vi "DMM Configuration.vi"(8 "error in (no error)":errorcluster, 11 "Node Ptr":T1 format="%.0x") -> (0 "error out":errorcluster)   [LabVIEW 2016, in "DMM-SWITCH-ScanList System Explorer.lvlib"]
uses:
  DMM-SWITCH-ScanList System Explorer.lvlib
  <vilib>/NI Veristand/Custom Device API/Custom Device Item Ref.ctl
  Configuration Controls/DMM Temp.ctl
  <instrlib>/niDMM/nidmm.llb/niDMM Transducer Type.ctl
  <instrlib>/niDMM/nidmm.llb/niDMM Thermocouple Type.ctl
  <instrlib>/niDMM/nidmm.llb/niDMM RTD Type.ctl
  <instrlib>/niDMM/nidmm.llb/niDMM Thermistor Type.ctl
  <instrlib>/niDMM/nidmm.llb/niDMM Function.ctl
  Shared/Constants.vi
  <vilib>/NI Veristand/Custom Device API/Get Item Property (U16).vi
  <vilib>/NI Veristand/Custom Device API/Get Item Property (Double).vi
  <vilib>/NI Veristand/Custom Device API/Get Item Property (String).vi
  <vilib>/NI Veristand/Custom Device API/Get Item Property (Variant).vi
  <vilib>/NI Veristand/Custom Device API/Set Item Property (String).vi
  <vilib>/NI Veristand/Custom Device API/Set Item Property (Double).vi
  <vilib>/NI Veristand/Custom Device API/Set Item Property (Variant).vi
  <vilib>/NI Veristand/Custom Device API/Set Item Property (U16).vi
  <vilib>/NI Veristand/Custom Device API/Custom Device API.lvlib
  Shared/DMM-SWITCH-ScanList Shared.lvlib
panel:
  in  "Temp3":dbl
  in  "Temp2":u16(ring)
  in  "Transducer":u16(ring)
  in  "Range":u16(ring)
  in  "Resolution in Digits":u16(ring)
  in  "Measurements":u16(ring)
  in  "DMM Resource Name":string
  in  "Header":cluster{"Section Name":string}={"Section Name"="Custom Device Item Settings"}
  in  "Description":string
  in  "Name":string
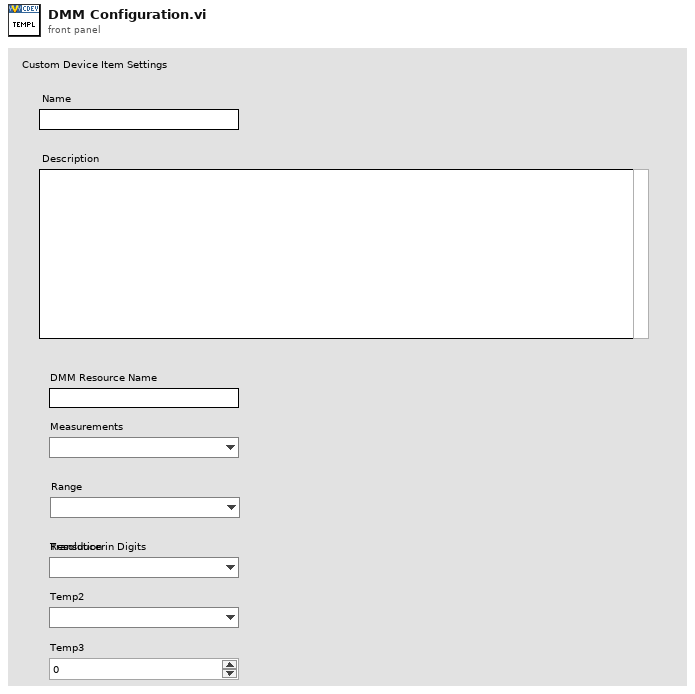
[diagram p1: front panel]
types:
  T1 = typedef "Custom Device API.lvlib/Custom Device Item Ref.ctl" = u64
  T2 = typedef "DMM-SWITCH-ScanList System Explorer.lvlib/DMM Temp.ctl" = cluster{"DMM Temp - Transducer Type":T3, "DMM Temp - Thermocouple Type":T4, "DMM Temp - Fixed Reference Junction":dbl, "DMM Temp - RTD Type":T5, "DMM Temp - RTD Resistance":dbl, "DMM Temp - Thermistor Type":T6, "DMM Temp - RTD A":dbl, "DMM Temp - RTD B":dbl, "DMM Temp - RTD C":dbl, "DMM Temp - Thermistor A":dbl, "DMM Temp - Thermistor B":dbl, "DMM Temp - Thermistor C":dbl}
  T3 = typedef "niDMM Transducer Type.ctl" = i32
  T4 = typedef "niDMM Thermocouple Type.ctl" = i32
  T5 = typedef "niDMM RTD Type.ctl" = enum16{"Custom", "Pt3750", "Pt3851", "Pt3911", "Pt3916", "Pt3920", "Pt3928"}
  T6 = typedef "niDMM Thermistor Type.ctl" = enum16{"Custom", "44004", "44006", "44007"}
  T7 = typedef "Custom Device API.lvlib/Custom Device Item Info.ctl" = cluster{"Name":string, "Is Channel":bool, "GUID":string, "Is Waveform":bool}
  T8 = cluster{"Measurements":refnum<vi>, "Range":refnum<vi>, "Resolution in Digits":refnum<vi>, "Transducer":refnum<vi>, "Temp2":refnum<vi>, "Temp3":refnum<vi>}
  T9 = typedef "niDMM Function.ctl" = enum16{"DC Volts", "AC Volts", "DC Current", "AC Current", "2-wire Resistance", "4-wire Resistance", "Diode", "Frequency", "Period", "AC Volts DC Coupled", "Capacitance", "Inductance", "Temperature"}
  T10 = typedef "Custom Device API.lvlib/Custom Device Commands.ctl" = enum16{"Default", "Item renamed", "Shutdown", "Dynamic button pressed"}
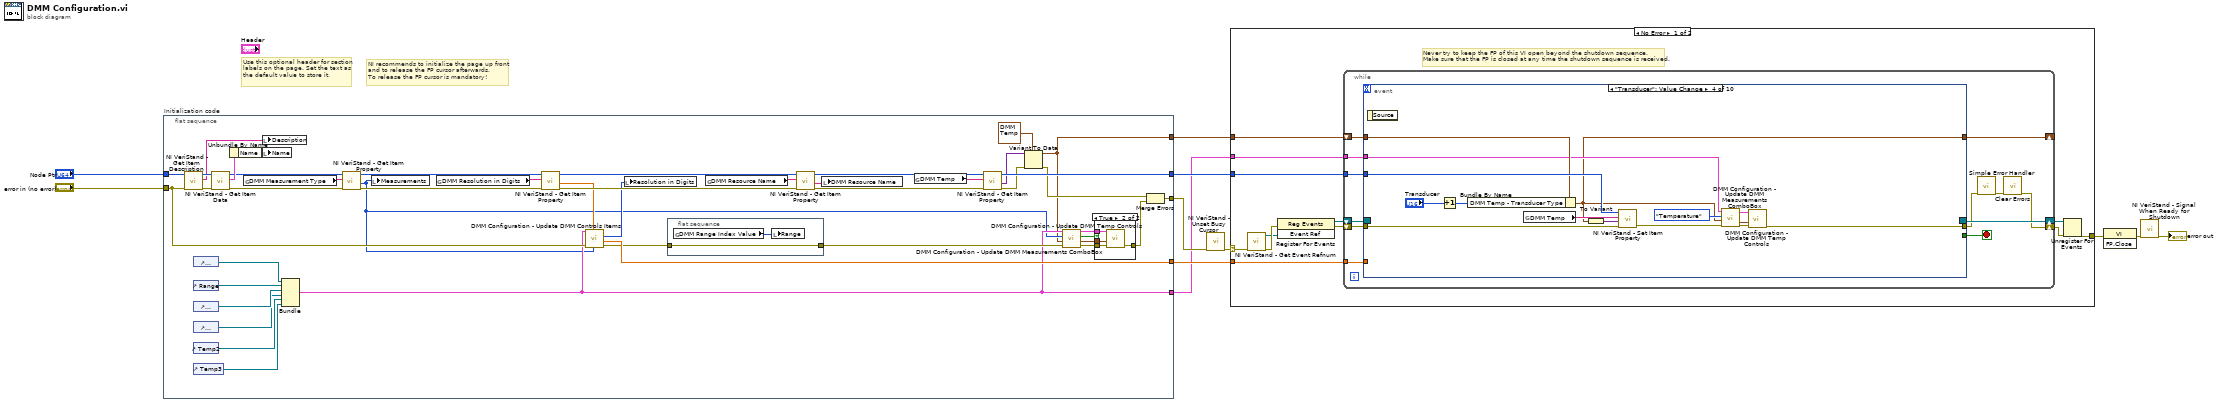
[diagram p0: block diagram]
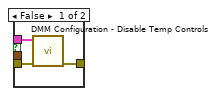
[diagram p2: hidden frame]
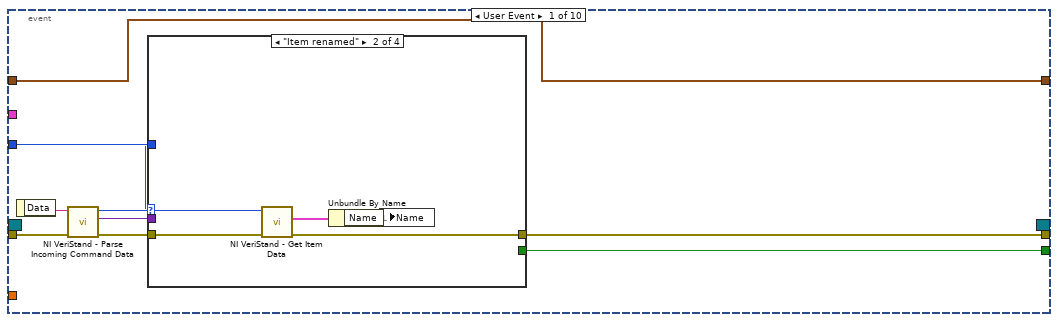
[diagram p3: hidden frame]
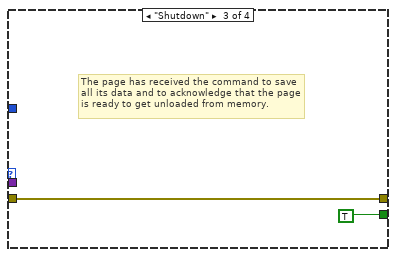
[diagram p5: hidden frame]
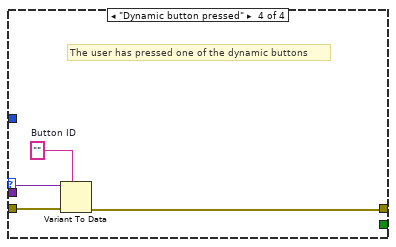
[diagram p6: hidden frame]
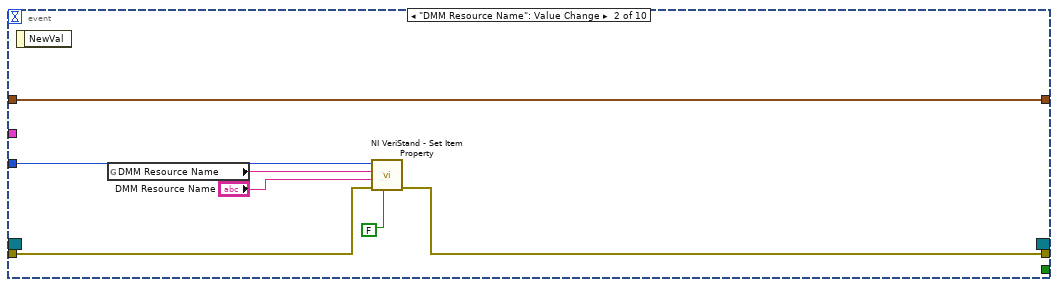
[diagram p7: hidden frame]
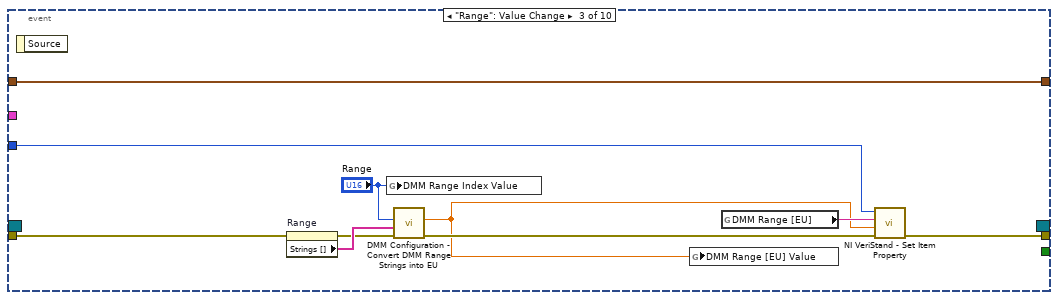
[diagram p8: hidden frame]
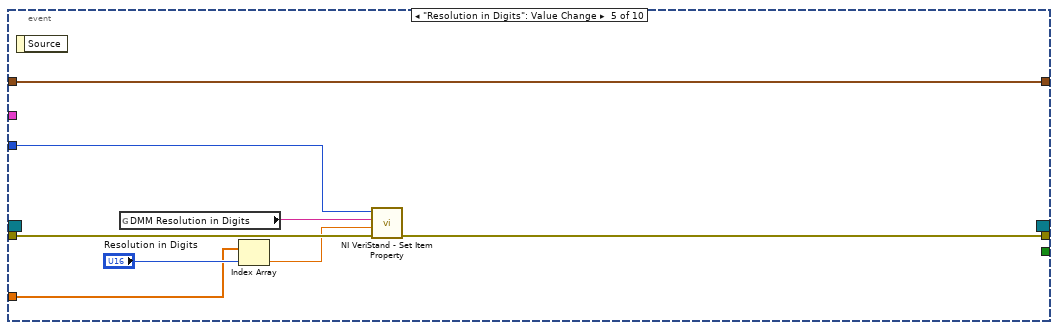
[diagram p9: hidden frame]
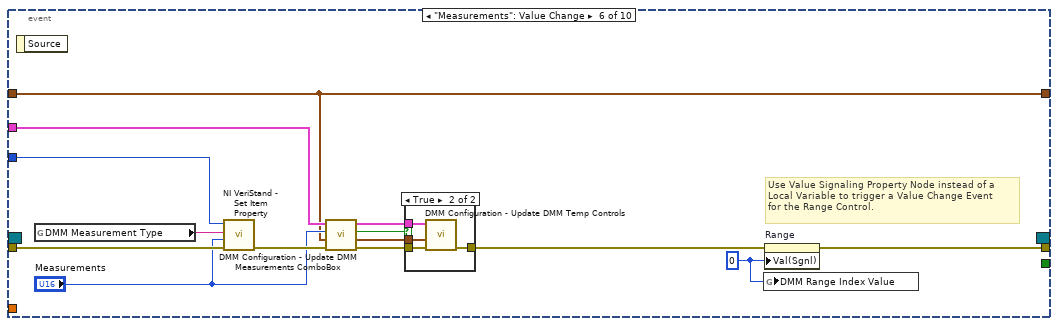
[diagram p10: hidden frame]
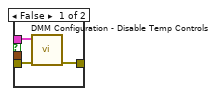
[diagram p11: hidden frame]
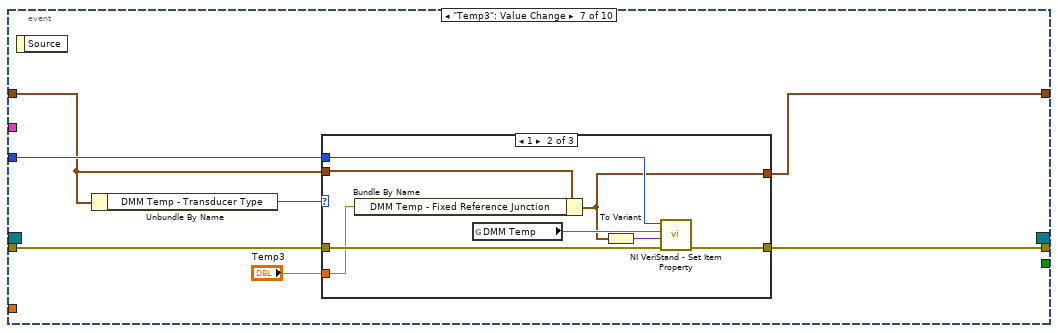
[diagram p12: hidden frame]
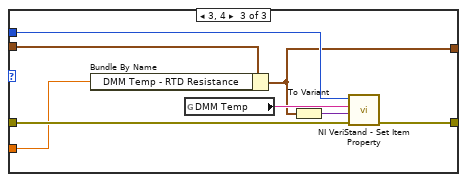
[diagram p14: hidden frame]
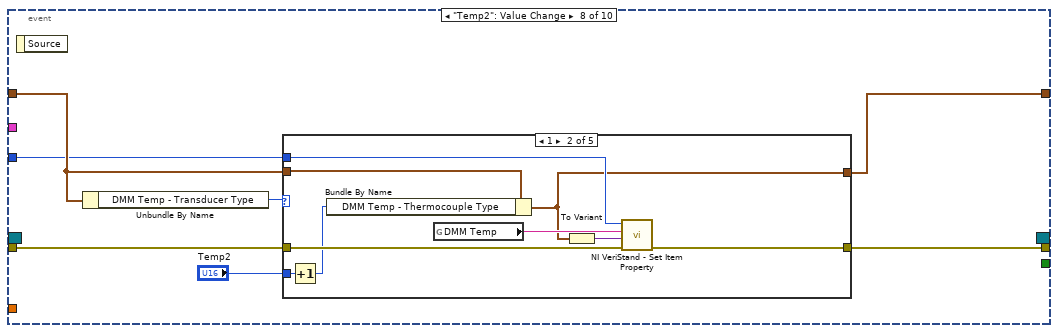
[diagram p15: hidden frame]
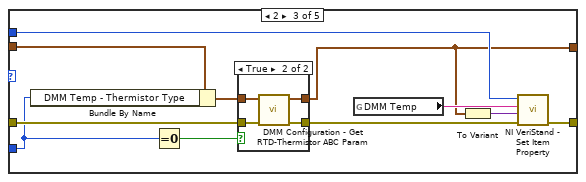
[diagram p17: hidden frame]
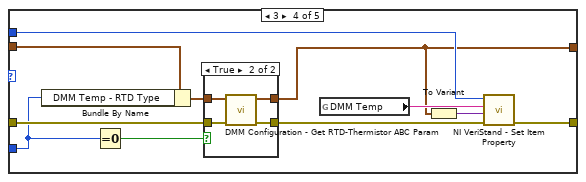
[diagram p19: hidden frame]
diagram:
  # "Use this optional header for section labels on the page. Set the text as the default value to store it."
  # "NI recommends to initialize the page up front\nand to release the FP cursor afterwards.\nTo release the FP cursor is mandatory!"
  n1 = flat-sequence "Initialization code" {
    tunnel: "error in (no error)" -> [w39]
    tunnel: "Node Ptr" -> [w55]
    tunnel: [w43] -> w7
    tunnel: [w25] -> w4
    tunnel: [w36] -> w3
    tunnel: [w17] -> w2
    tunnel: [w13] -> w1
    frame #0 {
      n2 = call <vilib>:"NI VeriStand - Get Item Description.vi"("error in (no error)"=w39, "Item Ref in"=w55) -> ("error out"=w53:errorcluster, "Description"=w54:string, "Item Ref out"=w56:T1)  [unwired: 7 out]
      n3 = control-ref of="Measurements"() -> (w29:refnum<vi>)
      n4 = control-ref of="Range"() -> (w34:refnum<vi>)
      n5 = control-ref of="Resolution in Digits"() -> (w33:refnum<vi>)
      n6 = control-ref of="Transducer"() -> (w31:refnum<vi>)
      n7 = control-ref of="Temp2"() -> (w30:refnum<vi>)
      n8 = control-ref of="Temp3"() -> (w32:refnum<vi>)
      n9 = call <vilib>:"NI VeriStand - Get Item Data.vi"("error in (no error)"=w53, "Item Ref in"=w56) -> ("error out"=w50:errorcluster, "Item Info"=w52:T7, "Item Ref out"=w49:T1)  [unwired: 7 out]
      n10 = Unbundle By Name(w52) -> ("Name"=w51:string)
      n11 = global read "Constants.vi" "DMM Measurement Type"() -> (w42:string)
      n12 = local write "Description"(w54) -> ()
      n13 = local write "Name"(w51) -> ()
      n14 = Bundle("Measurements"=w29, "Range"=w34, "Resolution in Digits"=w33, "Transducer"=w31, "Temp2"=w30, "Temp3"=w32) -> (w17:T8)  [unwired: 1 in]
      n15 = call-poly <vilib>:"NI VeriStand - Get Item Property.vi"("error in (no error)"=w50, "Property Name"=w42, "Item Ref in"=w49) -> ("error out"=w47:errorcluster, "Value"=w14:u16, "Item Ref out"=w48:T1)  [unwired: 5 in, 1 out]
      n16 = local write "Measurements"(w14) -> ()
      n17 = global read "Constants.vi" "DMM Resolution in Digits"() -> (w45:string)
      n18 = call-poly <vilib>:"NI VeriStand - Get Item Property.vi"("error in (no error)"=w47, "Property Name"=w45, "Item Ref in"=w48) -> ("error out"=w41:errorcluster, "Value"=w38:dbl, "Item Ref out"=w40:T1)  [unwired: 5 in, 1 out]
      n19 = call "DMM Configuration - Update DMM Controls Items.vi"("Measurement In"=w14, "Resolution in Digits Saved Value"=w38, "error in (no error)"=w39, "Measurement Controls Refs"=w17) -> ("error out"=w35:errorcluster, "Resolution in Digits Array Out"=w36:dbl[], "Resolution in Digits Index"=w37:i32)  [unwired: 5 in]
      n20 = local write "Resolution in Digits"(w37) -> ()
      n21 = flat-sequence {
        tunnel: w35 -> [w64]
        tunnel: [w64] -> w20
        frame #0 {
          n22 = global read "Constants.vi" "DMM Range Index Value"() -> (w65:u16)
          n23 = local write "Range"(w65) -> ()
        }
      }
      n24 = global read "Constants.vi" "DMM Resource Name"() -> (w44:string)
      n25 = call-poly <vilib>:"NI VeriStand - Get Item Property.vi"("error in (no error)"=w41, "Property Name"=w44, "Item Ref in"=w40) -> ("error out"=w27:errorcluster, "Value"=w46:string, "Item Ref out"=w26:T1)  [unwired: 5 in, 1 out]
      n26 = local write "DMM Resource Name"(w46) -> ()
      n27 = global read "Constants.vi" "DMM Temp"() -> (w28:string)
      n28 = call-poly <vilib>:"NI VeriStand - Get Item Property.vi"("error in (no error)"=w27, "Property Name"=w28, "Item Ref in"=w26) -> ("error out"=w24:errorcluster, "Value"=w22:variant, "Item Ref out"=w25:T1)  [unwired: 5 in, 1 out]
      n29 = Variant To Data(error in=w24, type=T2 {"DMM Temp - Transducer Type"=1, "DMM Temp - Thermocouple Type"=6, "DMM Temp - Fixed Reference Junction"=25.0, "DMM Temp - RTD Type"=enum."Pt3851", "DMM Temp - RTD Resistance"=100.0, "DMM Temp - Thermistor Type"=enum."44006", "DMM Temp - RTD A"=0.0039083, "DMM Temp - RTD B"=-5.775e-07, "DMM Temp - RTD C"=-4.183e-12, "DMM Temp - Thermistor A"=0.0010295, "DMM Temp - Thermistor B"=0.0002391, "DMM Temp - Thermistor C"=1.568e-07} ("DMM Temp - Value"), Variant=w22) -> (data=w13:T2, error out=w21:errorcluster)
      n30 = call "DMM Configuration - Update DMM Measurements ComboBox.vi"("error in (no error)"=w20, "DMM Temp - Value In"=w13, "Measurement In"=w14, "Measurement Controls Refs In"=w17) -> ("error out"=w19:errorcluster, "DMM Temp - Value Out"=w12:T2, "Temp Meas?"=w16:bool, "Measurement Controls Refs Out"=w15:T8)  [unwired: 4 in]
      n31 = case shown="True" w16 {
        tunnel: w15 -> [w59 w63]
        tunnel: w12 -> [_ w62]
        tunnel: w19 -> [w58 w61]
        tunnel: [w57 w60] -> w18
        frame False {
          n32 = call "DMM Configuration - Disable Temp Controls.vi"("error in (no error)"=w58, "Measurement Controls Refs"=w59) -> ("error out"=w57:errorcluster)  [unwired: 9 in]
        }
        frame True {
          n33 = call "DMM Configuration - Update DMM Temp Controls.vi"("error in (no error)"=w61, "DMM Temp - Value"=w62, "Measurement Controls Refs"=w63) -> ("error out"=w60:errorcluster)  [unwired: 8 in]
        }
      }
      n34 = Merge Errors(w21, w18) -> (w43:errorcluster)
    }
  }
  n35 = call <vilib>:"NI VeriStand - Unset Busy Cursor.vi"("error in (no error)"=w7) -> ("error out"=w6:errorcluster)  [unwired: 10 out]
  n36 = case shown="No Error" w6 {
    selector: w6 -> [w69 w278]
    tunnel: [w74 w276] -> w11
    tunnel: w4 -> [w70 _]
    tunnel: w3 -> [w68 _]
    tunnel: w2 -> [w67 _]
    tunnel: w1 -> [w66 _]
    frame No Error {
      # "Never try to keep the FP of this VI open beyond the shutdown sequence.\nMake sure that the FP is closed at any time the shutdown sequence is received."
      n37 = call <vilib>:"NI VeriStand - Get Event Refnum.vi"("error in (no error)"=w69) -> ("error out"=w77:errorcluster, "Event Ref"=w73:refnum<user-event>)  [unwired: 9 out]
      n38 = register-events(error in=w77, w73) -> (reference out=w71:refnum<event-registration>, error out=w72:errorcluster)  [unwired: 1 in]
      n39 = while {
        tunnel: w70 -> [w85]
        shift-right: [w82] -> w75
        shift-left: w72 -> [w88]
        shift-right: [w89] -> w76
        shift-left: w71 -> [w87]
        tunnel: w68 -> [w81]
        tunnel: w67 -> [w80]
        shift-right: [w78] -> _
        shift-left: w66 -> [w79]
        stop <- w86 stop-if-true
        n40 = event shown="[3] \"Transducer\": Value Change" {
          selector: w87 -> [_ _ _ _ _ _ _ _ _ _]
          dyn-events: [_ _ _ _ _ _ _ _ _ _] -> w89
          timeout: _ -> [_ _ _ _ _ _ _ _ _ _]
          tunnel: w88 -> [w98 w116 w125 w141 w149 w164 w178 w200 w270 w274]
          tunnel: [w94 _ _ _ _ _ _ _ _ _] -> w86
          tunnel: [w93 w115 w127 w137 w148 w161 w177 w199 w269 w273] -> w84
          tunnel: w85 -> [w92 w117 w124 w140 w150 w159 w175 w201 w268 w275]
          tunnel: w81 -> [_ _ _ _ w144 _ _ _ _ _]
          tunnel: w80 -> [_ _ _ w134 _ w157 _ _ _ _]
          tunnel: w79 -> [w90 w111 w118 w139 w143 w152 w173 w203 w266 w271]
          tunnel: [w90 w111 w118 w129 w143 w152 w172 w198 w266 w271] -> w78
          event User Event {
            n41 = event-data() -> ("Data"=w97:string)  [unwired: 1 out]
            n42 = call <vilib>:"NI VeriStand - Parse Incoming Command Data.vi"("error in (no error)"=w98, "Incoming data"=w97) -> ("error out"=w96:errorcluster, "Outgoing data"=w91:variant, "Action"=w95:T10)  [unwired: 7 out]
            n43 = case shown="\"Item renamed\"" w95 {
              tunnel: w96 -> [w99 w104 w105 w110]
              tunnel: [_ _ TRUE _] -> w94
              tunnel: [w99 w101 w105 w107] -> w93
              tunnel: w92 -> [_ w103 _ _]
              tunnel: w91 -> [_ _ _ w109]
              frame "Default", Default {
              }
              frame "Item renamed" {
                n44 = call <vilib>:"NI VeriStand - Get Item Data.vi"("error in (no error)"=w104, "Item Ref in"=w103) -> ("error out"=w101:errorcluster, "Item Info"=w102:T7)  [unwired: 8 out]
                n45 = Unbundle By Name(w102) -> ("Name"=w100:string)
                n46 = local write "Name"(w100) -> ()
              }
              frame "Shutdown" {
                # "The page has received the command to save all its data and to acknowledge that the page is ready to get unloaded from memory."
              }
              frame "Dynamic button pressed" {
                w108 = ""  # Button ID
                # "The user has pressed one of the dynamic buttons"
                n47 = Variant To Data(error in=w110, type=w108, Variant=w109) -> (error out=w107:errorcluster)  [unwired: 1 out]
              }
            }
          }
          event "DMM Resource Name": Value Change {
            n48 = event-data() -> ()  [unwired: 2 out]
            n49 = global read "Constants.vi" "DMM Resource Name"() -> (w112:string)
            n50 = call-poly <vilib>:"NI VeriStand - Set Item Property.vi"("Binary String (T)"=FALSE, "error in (no error)"=w116, "Value"="DMM Resource Name", "Property Name"=w112, "Item Ref in"=w117) -> ("error out"=w115:errorcluster)  [unwired: 4 in, 2 out]
          }
          event "Range": Value Change {
            n51 = event-data() -> ()  [unwired: 2 out]
            n52 = property on="Range" class="Ring (strict)"(error in=w125) -> (error out=w121:errorcluster, "Strings []"=w122:string[])  [unwired: 1 in, 1 out]
            n53 = global write "Constants.vi" "DMM Range Index Value"("Range") -> ()
            n54 = call "DMM Configuration - Convert DMM Range Strings into EU.vi"("error in (no error)"=w121, "DMM Range ComboBox Strings"=w122, "Dmm Range Index In"="Range") -> ("error out"=w120:errorcluster, "DMM Range [EU]"=w119:dbl)  [unwired: 7 in]
            n55 = global write "Constants.vi" "DMM Range [EU] Value"(w119) -> ()
            n56 = global read "Constants.vi" "DMM Range [EU]"() -> (w126:string)
            n57 = call-poly <vilib>:"NI VeriStand - Set Item Property.vi"("error in (no error)"=w120, "Value"=w119, "Property Name"=w126, "Item Ref in"=w124) -> ("error out"=w127:errorcluster)  [unwired: 5 in, 2 out]
          }
          event "Transducer": Value Change {
            n58 = event-data() -> ()  [unwired: 2 out]
            n59 = Increment(x="Transducer") -> (x+1=w135:u16)
            n60 = Bundle By Name(cluster=w139, "DMM Temp - Transducer Type"=w135) -> (w129:T2)
            n61 = global read "Constants.vi" "DMM Temp"() -> (w142:string)
            n62 = To Variant(anything=w129) -> (Variant=w138:variant)
            n63 = call-poly <vilib>:"NI VeriStand - Set Item Property.vi"("error in (no error)"=w141, "Value"=w138, "Property Name"=w142, "Item Ref in"=w140) -> ("error out"=w131:errorcluster)  [unwired: 5 in, 2 out]
            n64 = call "DMM Configuration - Update DMM Measurements ComboBox.vi"("error in (no error)"=w131, "DMM Temp - Value In"=w129, "Measurement In"=niDMM_Function."Temperature", "Measurement Controls Refs In"=w134) -> ("error out"=w130:errorcluster, "DMM Temp - Value Out"=w128:T2, "Measurement Controls Refs Out"=w133:T8)  [unwired: 4 in, 1 out]
            n65 = call "DMM Configuration - Update DMM Temp Controls.vi"("error in (no error)"=w130, "DMM Temp - Value"=w128, "Measurement Controls Refs"=w133) -> ("error out"=w137:errorcluster)  [unwired: 8 in]
          }
          event "Resolution in Digits": Value Change {
            n66 = event-data() -> ()  [unwired: 2 out]
            n67 = global read "Constants.vi" "DMM Resolution in Digits"() -> (w147:string)
            n68 = Index Array(array=w144, index="Resolution in Digits") -> (element=w146:dbl)
            n69 = call-poly <vilib>:"NI VeriStand - Set Item Property.vi"("error in (no error)"=w149, "Value"=w146, "Property Name"=w147, "Item Ref in"=w150) -> ("error out"=w148:errorcluster)  [unwired: 5 in, 2 out]
          }
          event "Measurements": Value Change {
            w162 = 0
            # "Use Value Signaling Property Node instead of a \nLocal Variable to trigger a Value Change Event \nfor the Range Control."
            n70 = event-data() -> ()  [unwired: 2 out]
            n71 = global read "Constants.vi" "DMM Measurement Type"() -> (w163:string)
            n72 = call-poly <vilib>:"NI VeriStand - Set Item Property.vi"("error in (no error)"=w164, "Value"="Measurements", "Property Name"=w163, "Item Ref in"=w159) -> ("error out"=w160:errorcluster)  [unwired: 5 in, 2 out]
            n73 = call "DMM Configuration - Update DMM Measurements ComboBox.vi"("error in (no error)"=w160, "DMM Temp - Value In"=w152, "Measurement In"="Measurements", "Measurement Controls Refs In"=w157) -> ("error out"=w156:errorcluster, "DMM Temp - Value Out"=w151:T2, "Temp Meas?"=w154:bool, "Measurement Controls Refs Out"=w153:T8)  [unwired: 4 in]
            n74 = case shown="True" w154 {
              tunnel: w153 -> [w165 w171]
              tunnel: w151 -> [_ w170]
              tunnel: w156 -> [w167 w169]
              tunnel: [w166 w168] -> w155
              frame False {
                n75 = call "DMM Configuration - Disable Temp Controls.vi"("error in (no error)"=w167, "Measurement Controls Refs"=w165) -> ("error out"=w166:errorcluster)  [unwired: 9 in]
              }
              frame True {
                n76 = call "DMM Configuration - Update DMM Temp Controls.vi"("error in (no error)"=w169, "DMM Temp - Value"=w170, "Measurement Controls Refs"=w171) -> ("error out"=w168:errorcluster)  [unwired: 8 in]
              }
            }
            n77 = global write "Constants.vi" "DMM Range Index Value"(w162) -> ()
            n78 = property on="Range" class="Ring (strict)"(error in=w155, "Val(Sgnl)"=w162) -> (error out=w161:errorcluster)  [unwired: 1 in, 1 out]
          }
          event "Temp3": Value Change {
            n79 = event-data() -> ()  [unwired: 2 out]
            n80 = Unbundle By Name(w173) -> ("DMM Temp - Transducer Type"=w176:T3)
            n81 = case shown="1" w176 {
              tunnel: w173 -> [w179 w186 w194]
              tunnel: w175 -> [_ w185 w191]
              tunnel: w178 -> [w180 w184 w193]
              tunnel: [w180 w183 w192] -> w177
              tunnel: "Temp3" -> [_ w182 w190]
              tunnel: [w179 w181 w189] -> w172
              frame 0, Default {
              }
              frame 1 {
                n82 = Bundle By Name(cluster=w186, "DMM Temp - Fixed Reference Junction"=w182) -> (w181:T2)
                n83 = global read "Constants.vi" "DMM Temp"() -> (w188:string)
                n84 = To Variant(anything=w181) -> (Variant=w187:variant)
                n85 = call-poly <vilib>:"NI VeriStand - Set Item Property.vi"("error in (no error)"=w184, "Value"=w187, "Property Name"=w188, "Item Ref in"=w185) -> ("error out"=w183:errorcluster)  [unwired: 5 in, 2 out]
              }
              frame 3, 4 {
                n86 = Bundle By Name(cluster=w194, "DMM Temp - RTD Resistance"=w190) -> (w189:T2)
                n87 = global read "Constants.vi" "DMM Temp"() -> (w196:string)
                n88 = To Variant(anything=w189) -> (Variant=w195:variant)
                n89 = call-poly <vilib>:"NI VeriStand - Set Item Property.vi"("error in (no error)"=w193, "Value"=w195, "Property Name"=w196, "Item Ref in"=w191) -> ("error out"=w192:errorcluster)  [unwired: 5 in, 2 out]
              }
            }
          }
          event "Temp2": Value Change {
            n90 = event-data() -> ()  [unwired: 2 out]
            n91 = Unbundle By Name(w203) -> ("DMM Temp - Transducer Type"=w202:T3)
            n92 = case shown="1" w202 {
              tunnel: w203 -> [w204 w212 w223 w240 w257]
              tunnel: w201 -> [_ w211 w221 w238 w255]
              tunnel: w200 -> [w205 w210 w220 w235 w252]
              tunnel: [w205 w209 w222 w239 w256] -> w199
              tunnel: [w204 w208 w215 w236 w253] -> w198
              tunnel: "Temp2" -> [_ w207 w218 w233 w249]
              frame 0, Default {
              }
              frame 1 {
                n93 = Increment(x=w207) -> (x+1=w206:u16)
                n94 = Bundle By Name(cluster=w212, "DMM Temp - Thermocouple Type"=w206) -> (w208:T2)
                n95 = global read "Constants.vi" "DMM Temp"() -> (w214:string)
                n96 = To Variant(anything=w208) -> (Variant=w213:variant)
                n97 = call-poly <vilib>:"NI VeriStand - Set Item Property.vi"("error in (no error)"=w210, "Value"=w213, "Property Name"=w214, "Item Ref in"=w211) -> ("error out"=w209:errorcluster)  [unwired: 5 in, 2 out]
              }
              frame 2 {
                n98 = Bundle By Name(cluster=w223, "DMM Temp - Thermistor Type"=w218) -> (w216:T2)
                n99 = Equal To 0?(x=w218) -> (x = 0?=w217:bool)
                n100 = case shown="True" w217 {
                  tunnel: w220 -> [w226 w231]
                  tunnel: [w226 w230] -> w219
                  tunnel: w216 -> [w227 w229]
                  tunnel: [w227 w228] -> w215
                  frame False {
                  }
                  frame True {
                    n101 = call "DMM Configuration - Get RTD-Thermistor ABC Param.vi"("error in (no error)"=w231, "DMM Temp - Value In"=w229) -> ("error out"=w230:errorcluster, "DMM Temp - Value Out"=w228:T2)  [unwired: 8 in]
                  }
                }
                n102 = global read "Constants.vi" "DMM Temp"() -> (w225:string)
                n103 = To Variant(anything=w215) -> (Variant=w224:variant)
                n104 = call-poly <vilib>:"NI VeriStand - Set Item Property.vi"("error in (no error)"=w219, "Value"=w224, "Property Name"=w225, "Item Ref in"=w221) -> ("error out"=w222:errorcluster)  [unwired: 5 in, 2 out]
              }
              frame 3 {
                n105 = Bundle By Name(cluster=w240, "DMM Temp - RTD Type"=w233) -> (w237:T2)
                n106 = Equal To 0?(x=w233) -> (x = 0?=w232:bool)
                n107 = case shown="True" w232 {
                  tunnel: w237 -> [w244 w248]
                  tunnel: [w244 w247] -> w236
                  tunnel: w235 -> [w243 w246]
                  tunnel: [w243 w245] -> w234
                  frame False {
                  }
                  frame True {
                    n108 = call "DMM Configuration - Get RTD-Thermistor ABC Param.vi"("error in (no error)"=w246, "DMM Temp - Value In"=w248) -> ("error out"=w245:errorcluster, "DMM Temp - Value Out"=w247:T2)  [unwired: 8 in]
                  }
                }
                n109 = global read "Constants.vi" "DMM Temp"() -> (w242:string)
                n110 = To Variant(anything=w236) -> (Variant=w241:variant)
                n111 = call-poly <vilib>:"NI VeriStand - Set Item Property.vi"("error in (no error)"=w234, "Value"=w241, "Property Name"=w242, "Item Ref in"=w238) -> ("error out"=w239:errorcluster)  [unwired: 5 in, 2 out]
              }
              frame 4 {
                n112 = Bundle By Name(cluster=w257, "DMM Temp - RTD Type"=w249) -> (w254:T2)
                n113 = Equal To 0?(x=w249) -> (x = 0?=w250:bool)
                n114 = case shown="True" w250 {
                  tunnel: w254 -> [w261 w265]
                  tunnel: [w261 w264] -> w253
                  tunnel: w252 -> [w260 w263]
                  tunnel: [w260 w262] -> w251
                  frame False {
                  }
                  frame True {
                    n115 = call "DMM Configuration - Get RTD-Thermistor ABC Param.vi"("error in (no error)"=w263, "DMM Temp - Value In"=w265) -> ("error out"=w262:errorcluster, "DMM Temp - Value Out"=w264:T2)  [unwired: 8 in]
                  }
                }
                n116 = global read "Constants.vi" "DMM Temp"() -> (w259:string)
                n117 = To Variant(anything=w253) -> (Variant=w258:variant)
                n118 = call-poly <vilib>:"NI VeriStand - Set Item Property.vi"("error in (no error)"=w251, "Value"=w258, "Property Name"=w259, "Item Ref in"=w255) -> ("error out"=w256:errorcluster)  [unwired: 5 in, 2 out]
              }
            }
          }
          event "Name": Value Change {
            n119 = event-data() -> ()  [unwired: 2 out]
            n120 = call <vilib>:"NI VeriStand - Rename Custom Device Item.vi"("error in (no error)"=w270, "New Name"="Name", "Item Ref in"=w268) -> ("error out"=w269:errorcluster)  [unwired: 1 in, 7 out]
          }
          event "Description": Value Change {
            n121 = event-data() -> ()  [unwired: 2 out]
            n122 = call <vilib>:"NI VeriStand - Set Item Description.vi"("error in (no error)"=w274, "Description"="Description", "Item Ref in"=w275) -> ("error out"=w273:errorcluster)  [unwired: 8 out]
          }
        }
        n123 = call <vilib>:"Simple Error Handler.vi"("error in (no error)"=w84) -> ("error out"=w83:errorcluster)  [unwired: 1 in, 7 out]
        n124 = call <vilib>:"Clear Errors.vi"("error in (no error)"=w83) -> ("error out"=w82:errorcluster)  [unwired: 1 in, 5 out]
      }
      n125 = Unregister For Events(event registration refnum=w76, error in=w75) -> (error out=w74:errorcluster)
    }
    frame Error {
      n126 = call <vilib>:"Simple Error Handler.vi"("error in (no error)"=w278) -> ("error out"=w277:errorcluster)  [unwired: 1 in, 7 out]
      n127 = call <vilib>:"Clear Errors.vi"("error in (no error)"=w277) -> ("error out"=w276:errorcluster)  [unwired: 1 in, 5 out]
    }
  }
  n128 = invoke class="VI" method="FP.Close"(error in=w11) -> (error out=w10:errorcluster)  [unwired: 2 in, 2 out]
  n129 = call <vilib>:"NI VeriStand - Signal When Ready for Shutdown.vi"("error in (no error)"=w10) -> ("error out"=→"error out":errorcluster)  [unwired: 10 out]
